vi "ICM Convert Format to Array.vi"(11 "Format String":string) -> (3 "Format Array":string[](array[string]))   [LabVIEW 2018]
doc: "ICM Convert Format to Array.vi\n\n This VI is used to take a Format String and convert it to an array of format strings.\n\nThis VI was original part of the OSDS system.\n\nInstrument Communication Module Version 1.0\nSeptember, 2017 Original Code Consulting David Thomson\n www.originalcode.com"
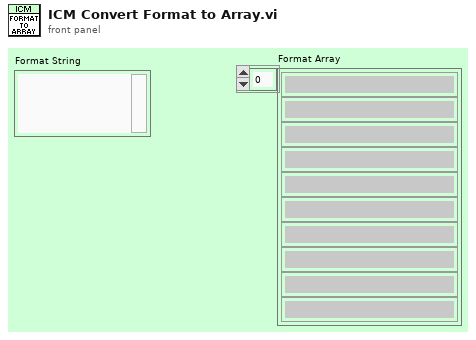
[diagram p1: front panel]
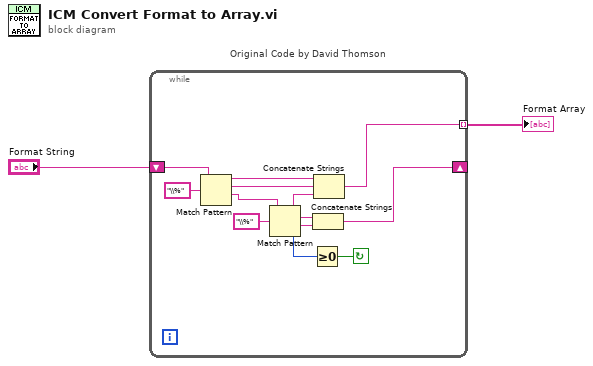
[diagram p0: block diagram]
diagram:
  n1 = while "Original Code by David Thomson" {
    shift-right: [w8] -> _
    shift-left: "Format String" -> [w14]
    tunnel: [w3] -> w2 mode=indexing
    stop <- w13 continue-if-true
    n2 = Match Pattern(string=w14, regular expression="\\%") -> (before substring=w7:string, match substring=w6:string, after substring=w5:string)  [unwired: 2 out]
    n3 = Match Pattern(string=w5, regular expression="\\%") -> (before substring=w4:string, match substring=w11:string, after substring=w12:string, offset past match=w9:i32)  [unwired: 1 out]
    n4 = Greater Or Equal To 0?(x=w9) -> (x >= 0?=w13:bool)
    n5 = Concatenate Strings(w11, w12) -> (w8:string)
    n6 = Concatenate Strings(w7, w6, w4) -> (w3:string)
  }
  "Format Array" <- w2
